vi "AddAssignedButtons_171213.vi"(10 "IndexOfTheIncreasedVaule":i32, 11 "KeyboardShortCutsArray":string[][](array[string])) -> (3 "KeyboardShortCutArray":string[][](array[string]))   [LabVIEW 2016]
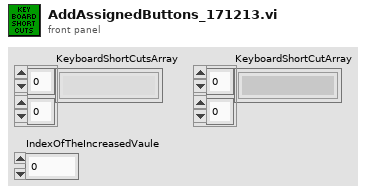
[diagram p1: front panel]
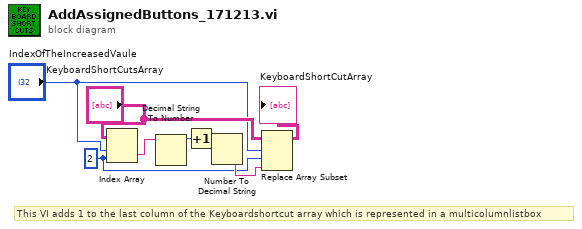
[diagram p0: block diagram]
diagram:
  w4 = 2 ("disabled index (col)")
  # "This VI adds 1 to the last column of the Keyboardshortcut array which is represented in a multicolumnlistbox"
  n1 = Index Array(array="KeyboardShortCutsArray", index (row)="IndexOfTheIncreasedVaule", index (col)=w4) -> (element=w1:string)
  n2 = Decimal String To Number(string=w1) -> (number=w2:i32)  [unwired: 2 in, 1 out]
  n3 = Increment(x=w2) -> (x+1=w3:i32)
  n4 = Number To Decimal String(number=w3) -> (decimal integer string=w6:string)  [unwired: 1 in]
  n5 = Replace Array Subset(array="KeyboardShortCutsArray", new element=w6, index (row)="IndexOfTheIncreasedVaule", index (col)=w4) -> (→"KeyboardShortCutArray":string[][])
